vi "Initialize.vi"(4 "Shutter Enable":bool[](array[boolean]), 5 "Duty cycle":dbl=1.0, 6 "ALEX":bool, 7 "Interval (ms)":dbl, 8 "error in (no error)":errorcluster, 9 "Shutter Lines":string[](array[string]), 10 "Sync Line":string, 11 "Synchronization Device in":refnum<class "Synchronization Device.lvclass">) -> (0 "error out":errorcluster, 3 "Synchronization Device out":refnum<class "Synchronization Device.lvclass">)   [LabVIEW 2018, in "Synchronization Device.lvlib" / "Synchronization Device.lvclass"]
uses:
  Synchronization Device.lvclass
  Synchronization Device.lvclass/Synchronization Device.ctl
  <vilib>/DAQmx/create/channels.llb/DAQmx Create Channel (DO-Digital Output).vi
  <resource>/objmgr/daqmx.rc
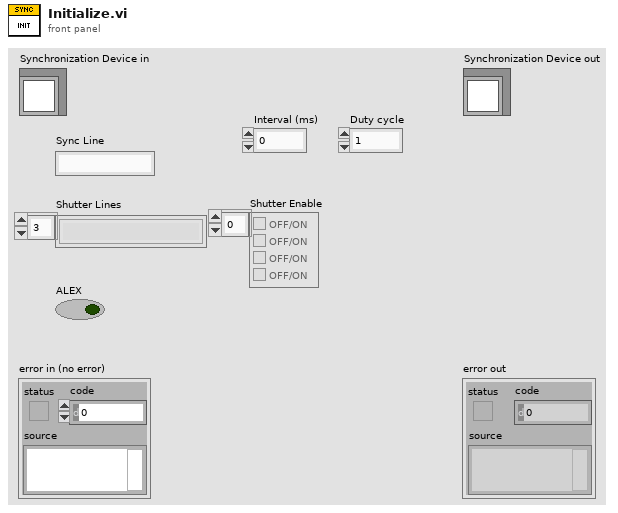
[diagram p1: front panel]
types:
  T1 = cluster{"Interval (ms)":dbl, "ALEX":bool, "Shutter Enable":bool[], "Stream":bool, "Duty Cycle":dbl, "Timelapse Interval (s)":u32}
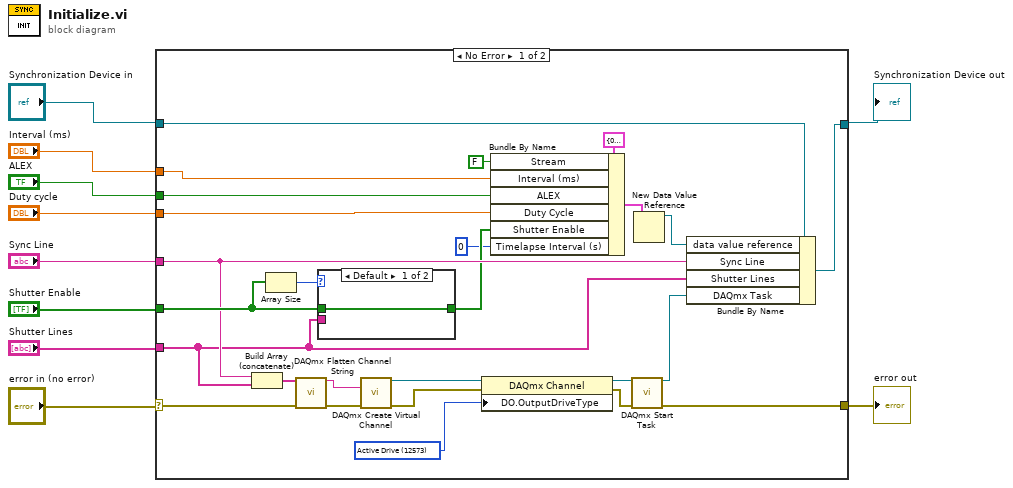
[diagram p0: block diagram]
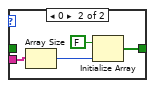
[diagram p2: hidden frame]
diagram:
  n1 = case shown="No Error" "error in (no error)" {
    selector: "error in (no error)" -> [w20 w43]
    tunnel: [w21 w43] -> w9
    tunnel: [w35 w42] -> w7
    tunnel: "Synchronization Device in" -> [w36 w42]
    tunnel: "Sync Line" -> [w19 _]
    tunnel: "Interval (ms)" -> [w33 _]
    tunnel: "Shutter Lines" -> [w18 _]
    tunnel: "ALEX" -> [w32 _]
    tunnel: "Shutter Enable" -> [w30 _]
    tunnel: "Duty cycle" -> [w14 _]
    frame No Error {
      w22 = 12573 items=["Active Drive"=12573, "Open Collector"=12574] ("DO.OutputDriveType")
      n2 = Build Array (concatenate)(w19, w18) -> (w25:string[])
      n3 = Array Size(array=w30) -> (size(s)=w31:i32)
      n4 = call <vilib>:"DAQmx Flatten Channel String.vi"("names in"=w25, "error in"=w20) -> ("names out"=w24:string, "error out"=w23:errorcluster)  [unwired: 12 in]
      n5 = case shown="Default" w31 {
        tunnel: w18 -> [_ w40]
        tunnel: [w37 w38] -> w15
        tunnel: w30 -> [w37 _]
        frame Default {
        }
        frame 0 {
          n6 = Array Size(array=w40) -> (size(s)=w41:i32)
          n7 = Initialize Array(FALSE, w41) -> (w38:bool[])
        }
      }
      n8 = call-poly <vilib>:"DAQmx Create Virtual Channel.vi"("lines"=w24, "error in"=w23) -> ("task out"=w29:refnum<k21>, "error out"=w27:errorcluster)  [unwired: 12 in]
      n9 = property class="DAQmx Channel"(reference=w29, error in=w27, "DO.OutputDriveType"=w22) -> (reference out=w28:refnum<k21>, error out=w26:errorcluster)
      n10 = Bundle By Name(cluster=T1 {"Interval (ms)"=0.0, "ALEX"=FALSE, "Shutter Enable"=[], "Stream"=FALSE, "Duty Cycle"=0.0, "Timelapse Interval (s)"=0} ("input cluster"), "Stream"=FALSE, "Interval (ms)"=w33, "ALEX"=w32, "Duty Cycle"=w14, "Shutter Enable"=w15, "Timelapse Interval (s)"=u32 0) -> (w34:T1)
      n11 = call <vilib>:"DAQmx Start Task.vi"("task/channels in"=w28, "error in"=w26) -> ("task out"=w17:refnum<k21>, "error out"=w21:errorcluster)  [unwired: 12 in]
      n12 = New Data Value Reference(data value=w34) -> (data value reference=w13:refnum<data-value>)  [unwired: 1 in, 1 out]
      n13 = Bundle By Name(cluster=w36, "data value reference"=w13, "Sync Line"=w19, "Shutter Lines"=w18, "DAQmx Task"=w17) -> (w35:refnum<class "Synchronization Device.lvclass">)
    }
    frame Error {
    }
  }
  "error out" <- w9
  "Synchronization Device out" <- w7
